vi "Throw Existing Handler.vi"(8 "error in (no error)":errorcluster) -> (0 "error out":errorcluster)   [LabVIEW 2020, in "ExecAnchor.lvclass"]
uses:
  ExecAnchor.lvclass
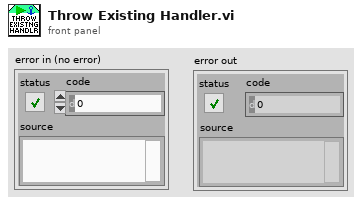
[diagram p1: front panel]
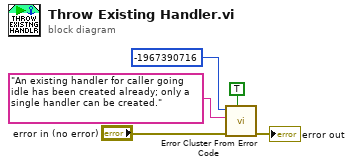
[diagram p0: block diagram]
diagram:
  n1 = call <vilib>:"Error Cluster From Error Code.vi"("show call chain? (False)"=TRUE, "error in (no error)"="error in (no error)", "error message (\"\")"="An existing handler for caller going idle has been created already; only a single handler can be created." ("error message (\"\")"), "error code (0)"=-1967390716) -> ("error out"=→"error out":errorcluster)  [unwired: 5 in]
